vi "Example Callback.vi"() -> ()   [LabVIEW 2013]
uses:
  C:/tf/play/labview/Tinkerforge.dll
  Tinkerforge.dll
panel:
  in  "stop":bool
  in  "uid":string="63oL6P"
  in  "port":i32=4223
  in  "host":string="localhost"
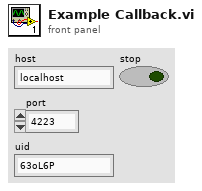
[diagram p1: front panel]
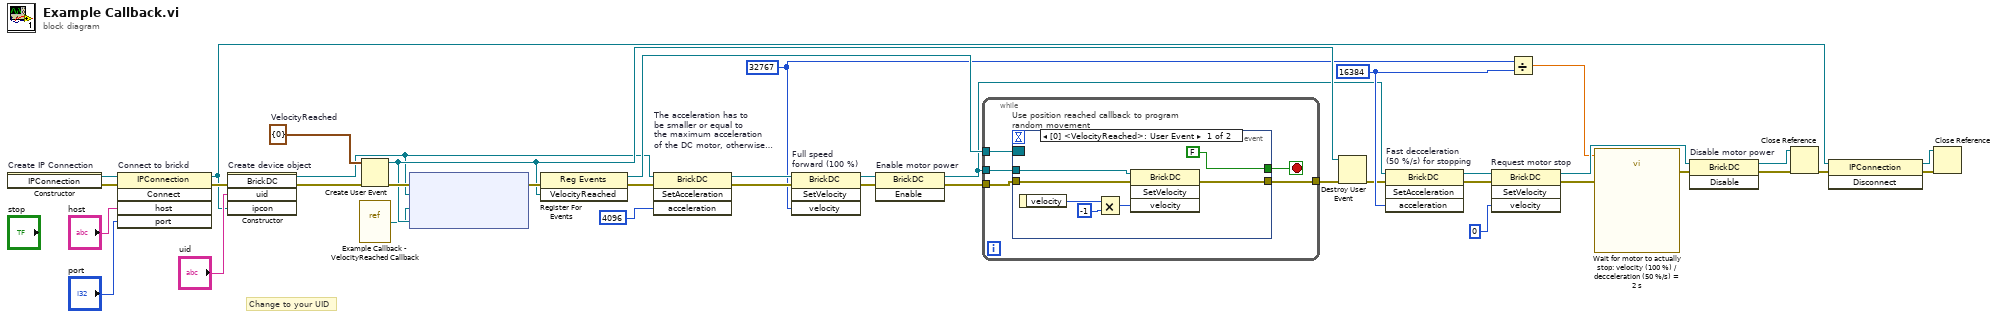
[diagram p0: block diagram]
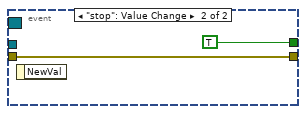
[diagram p2: hidden frame]
diagram:
  w6 = 16384 ("acceleration")
  w1 = i16 32767 ("velocity")
  w25 = cluster{"velocity":i16} {"velocity"=0}  # VelocityReached
  # "Change to your UID"
  n1 = constructor on="Create IP Connection" class="IPConnection"() -> (reference out=w39:refnum<k24>, error out=w14:errorcluster)  [unwired: 3 in, 1 out]
  n2 = invoke on="Connect to brickd" class="IPConnection" method="Connect"(reference=w39, error in=w14, "host"="host", "port"="port") -> (reference out=w32:refnum<k24>, error out=w35:errorcluster)  [unwired: 1 in, 3 out]
  n3 = constructor on="Create device object" class="BrickDC"(error in=w35, "uid"="uid", "ipcon"=w32) -> (reference out=w23:refnum<k24>, error out=w24:errorcluster)  [unwired: 2 in, 3 out]
  n4 = vi-ref "Example Callback - VelocityReached Callback.vi"() -> ("vi reference"=w19:refnum<vi>)
  n5 = Create User Event(user event datatype=w25, error in=w24) -> (user event=w26:refnum<user-event>, error out=w30:errorcluster)
  n6 = node ("Register Event Callback")(w30, w23, w19, w26) -> (w29:errorcluster)  [unwired: 1 in, 1 out]
  n7 = register-events(error in=w29, w26) -> (reference out=w28:refnum<event-registration>, error out=w22:errorcluster)  [unwired: 1 in]
  n8 = invoke on="The acceleration has to\nbe smaller or equal to\nthe maximum acceleration\nof the DC motor, otherwise\nVelocityReached will be\ncalled too early.\nSlow acceleration (12.5 %/s)" class="BrickDC" method="SetAcceleration"(reference=w23, error in=w22, "acceleration"=4096) -> (reference out=w18:refnum<k24>, error out=w17:errorcluster)  [unwired: 1 in, 2 out]
  n9 = invoke on="Full speed \nforward (100 %)" class="BrickDC" method="SetVelocity"(reference=w18, error in=w17, "velocity"=w1) -> (reference out=w15:refnum<k24>, error out=w16:errorcluster)  [unwired: 1 in, 2 out]
  n10 = invoke on="Enable motor power" class="BrickDC" method="Enable"(reference=w15, error in=w16) -> (reference out=w5:refnum<k24>, error out=w21:errorcluster)  [unwired: 1 in, 1 out]
  n11 = while {
    tunnel: w28 -> [w44]
    tunnel: [w43] -> w27
    tunnel: w21 -> [w42]
    tunnel: w5 -> [w41]
    stop <- w40 stop-if-true
    n12 = event "Use position reached callback to program random movement" shown="[0] <VelocityReached>: User Event" {
      selector: w44 -> [_ _]
      dyn-events: _ -> [_ _]
      timeout: _ -> [_ _]
      tunnel: [w48 w52] -> w43
      tunnel: w42 -> [w51 w52]
      tunnel: w41 -> [w50 _]
      tunnel: [FALSE TRUE] -> w40
      event User Event {
        n13 = event-data() -> ("velocity"=w47:i16)  [unwired: 1 in]
        n14 = Multiply(x=w47, y=i16 -1) -> (x*y=w46:i16)
        n15 = invoke class="BrickDC" method="SetVelocity"(reference=w50, error in=w51, "velocity"=w46) -> (error out=w48:errorcluster)  [unwired: 1 in, 3 out]
      }
      event "stop": Value Change {
        n16 = event-data() -> ()  [unwired: 1 in, 1 out]
      }
    }
  }
  n17 = Destroy User Event(user event=w26, error in=w27) -> (error out=w2:errorcluster)
  n18 = invoke on="Fast decceleration\n(50 %/s) for stopping" class="BrickDC" method="SetAcceleration"(reference=w5, error in=w2, "acceleration"=w6) -> (reference out=w13:refnum<k24>, error out=w12:errorcluster)  [unwired: 1 in, 2 out]
  n19 = invoke on="Request motor stop" class="BrickDC" method="SetVelocity"(reference=w13, error in=w12, "velocity"=i16 0) -> (reference out=w8:refnum<k24>, error out=w10:errorcluster)  [unwired: 1 in, 2 out]
  n20 = Divide(x=w1, y=w6) -> (x/y=w7:dbl)
  n21 = call "Wait for motor to actually stop: velocity (100 %) / decceleration (50 %/s) = 2 s"("error in (no error)"=w10, "Delay Time (s)"=w7) -> ("error out"=w9:errorcluster)  [unwired: 9 in]
  n22 = invoke on="Disable motor power" class="BrickDC" method="Disable"(reference=w8, error in=w9) -> (reference out=w4:refnum<k24>, error out=w3:errorcluster)  [unwired: 1 in, 1 out]
  n23 = Close Reference(reference=w4, error in (no error)=w3) -> (error out=w34:errorcluster)
  n24 = invoke class="IPConnection" method="Disconnect"(reference=w32, error in=w34) -> (reference out=w31:refnum<k24>, error out=w33:errorcluster)  [unwired: 1 in, 1 out]
  n25 = Close Reference(reference=w31, error in (no error)=w33) -> ()  [unwired: 1 out]
